vi "AGCxxx Command UnitS.vi"(7 "error in (no error)":errorcluster, 9 "unit (mBar)":enum16{"mBar", "Pascal", "Torr"}(ring), 10 "AGCxxx VISA Cluster":T1={"VISA resource name"="", "VISA Timeout Value (1000 ms)"=1000, "Lock Timeout (1000 ms)"=1000, "MAX Channel (6)"=6}) -> (0 "error out":errorcluster, 1 "AGC Errno":i32, 3 "dup AGCxxx VISA Cluster":T1={"VISA resource name"="", "VISA Timeout Value (1000 ms)"=1000, "Lock Timeout (1000 ms)"=1000, "MAX Channel (6)"=6})   [LabVIEW 2014, in "AGCxxx - Driver.lvlib"]
doc: "Sets the units x, as in the SYSTEM menu.\n\n1 = mBar\n2 = Pascal\n3 = Torr\n\n! AGC Needs 10 Seconds to change the Unit !\n\n\nCopyright (C) \nGesellschaft f. Schwerionenforschung, GSI\nPlanckstr. 1\n64291 Darmstadt\nGermany\n\nContact: http://www-wnt.gsi.de/labview\n H.Brand@gsi.de\n\nThis program is free software; you can redistribute it and/or\nmodify it under the terms of the GNU General Public License\nas published by the Free Software Foundation; either version 2\nof the License, or (at your option) any later version.\n\nThis program is distributed in the hope that it will be useful,\nbut WITHOUT ANY WARRANTY; without even the implied warranty of\nMERCHANTABILITY or FITNESS FOR A PARTICULAR PURPOSE. See the\nGNU General Public License for more details (http://www.gnu.org)."
uses:
  AGCxxx - Driver.lvlib
  AGCxxx VISA Control.ctl
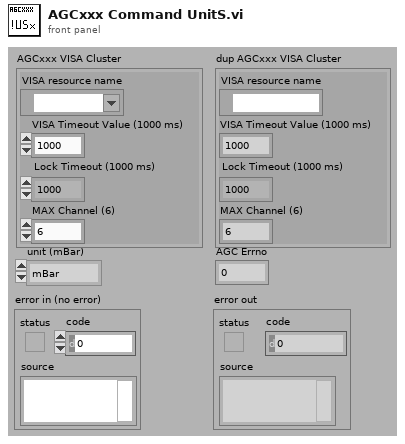
[diagram p1: front panel]
types:
  T1 = typedef "AGCxxx - Driver.lvlib/AGCxxx VISA Control.ctl" = cluster{"VISA resource name":refnum<visa-resource-name>, "VISA Timeout Value (1000 ms)":u32, "Lock Timeout (1000 ms)":u32, "MAX Channel (6)":i32}
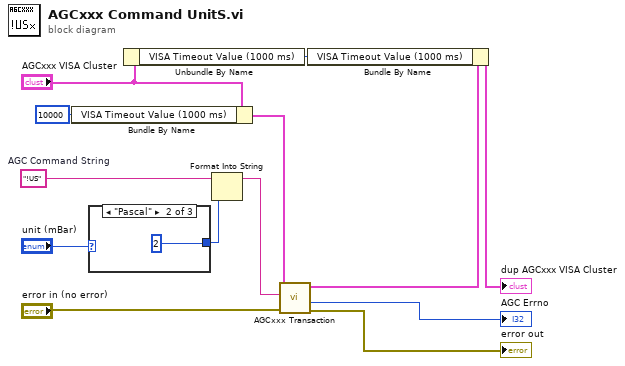
[diagram p0: block diagram]
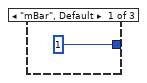
[diagram p2: hidden frame]
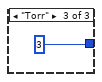
[diagram p3: hidden frame]
diagram:
  w10 = "!US"  # AGC Command String
  n1 = Bundle By Name(cluster="AGCxxx VISA Cluster", "VISA Timeout Value (1000 ms)"=u32 10000) -> (w6:T1)
  n2 = case shown="\"Pascal\"" "unit (mBar)" {
    tunnel: [1 2 3] -> w8
    frame "mBar", Default {
    }
    frame "Pascal" {
    }
    frame "Torr" {
    }
  }
  n3 = Unbundle By Name("AGCxxx VISA Cluster") -> ("VISA Timeout Value (1000 ms)"=w2:u32)
  n4 = Format Into String(initial string=w10, w8) -> (resulting string=w7:string)  [unwired: 2 in, 1 out]
  n5 = call "AGCxxx Transaction.vi"("error in (no error)"="error in (no error)", "AGC Command String"=w7, "AGCxxx VISA Cluster"=w6) -> ("error out"=→"error out":errorcluster, "AGC Errno"=→"AGC Errno":i32, "dup AGCxxx VISA Cluster"=w3:T1)  [unwired: 4 in, 1 out]
  n6 = Bundle By Name(cluster=w3, "VISA Timeout Value (1000 ms)"=w2) -> (→"dup AGCxxx VISA Cluster":T1)
